vi "GetWaveformChartReference.vi"(8 "error in":errorcluster, 11 "WFChart in":refnum<class "WaveformChart.lvclass">) -> (0 "error out":errorcluster, 1 "graph scale reference":refnum<vi>, 3 "WFChart out":refnum<class "WaveformChart.lvclass">)   [LabVIEW 2014, in "Raspberry Pi Compatible Compiler for LabVIEW.lvlib" / "WaveformChart.lvclass"]
uses:
  WaveformChart.lvclass
  Generic/Generic.lvclass
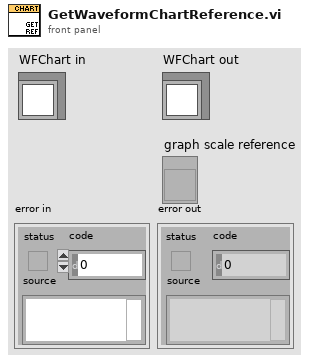
[diagram p1: front panel]
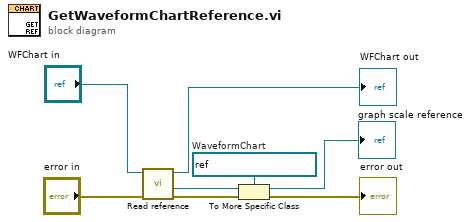
[diagram p0: block diagram]
diagram:
  w5 = refnum<vi> refnum  # WaveformChart
  n1 = call "Read reference.vi"("error in"="error in", "GObject in"="WFChart in") -> ("error out"=w6:errorcluster, "reference"=w7:refnum<vi>, "GObject out"=→"WFChart out":refnum<class "WaveformChart.lvclass">)  [unwired: 5 in]
  n2 = To More Specific Class(target class=w5, reference=w7, error in=w6) -> (specific class reference=→"graph scale reference":refnum<vi>, error out=→"error out":errorcluster)
